vi "Untitled 3.vi"() -> ()   [LabVIEW 2017]
uses:
  <vilib>/Analysis/baseanly.llb/Mean (DBL).vi
  <vilib>/Analysis/NI_AALBase.lvlib
panel:
  in  "Tempi":i32[](array[numeric])
  in  "i":i32
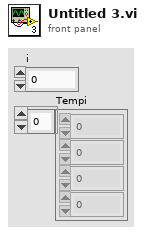
[diagram p1: front panel]
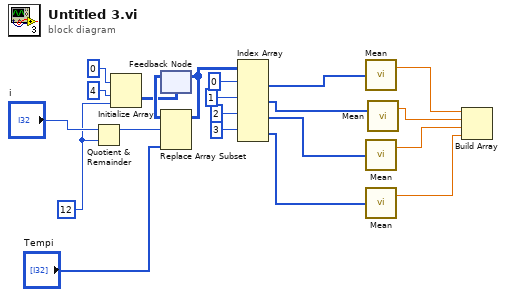
[diagram p0: block diagram]
diagram:
  w15 = 12 ("dimension size")
  n1 = Quotient & Remainder(x="i", y=w15) -> (x-y*floor(x/y)=w18:i32)  [unwired: 1 out]
  n2 = Initialize Array(0, 4 ("dimension size"), w15) -> (w20:i32[][])
  n3 = feedback #1(w20) -> (w21:i32[][])
  n4 = Replace Array Subset(array=w21, new element="Tempi", index (row)=w18) -> (w14:i32[][])  [unwired: 1 in]
  n5 = feedback-in #1(w14) -> ()
  n6 = Index Array(array=w14, index (row) #1=0 ("index (row)"), index (row) #2=1 ("index (row)"), index (row) #3=2 ("index (row)"), index (row) #4=3 ("index (row)")) -> (element #1=w9:i32[], element #2=w8:i32[], element #3=w7:i32[], element #4=w6:i32[])  [unwired: 4 in]
  n7 = call-poly <vilib>:"Mean.vi"("X"=w9) -> ("mean"=w5:dbl)  [unwired: 1 out]
  n8 = call-poly <vilib>:"Mean.vi"("X"=w7) -> ("mean"=w3:dbl)  [unwired: 1 out]
  n9 = call-poly <vilib>:"Mean.vi"("X"=w6) -> ("mean"=w2:dbl)  [unwired: 1 out]
  n10 = call-poly <vilib>:"Mean.vi"("X"=w8) -> ("mean"=w4:dbl)  [unwired: 1 out]
  n11 = Build Array(w5, w4, w3, w2) -> ()  [unwired: 1 out]
